vi "Validate Group Time.vi"(0 "Group time":u8) -> (2 "Group Time":u16, 3 "Warning":string, 4 "Frequency (Hz)":dbl)   [LabVIEW 2019]
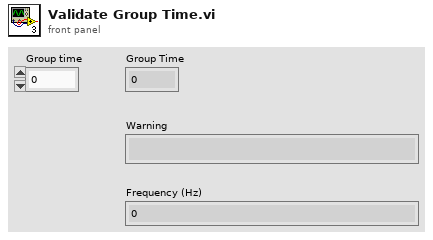
[diagram p1: front panel]
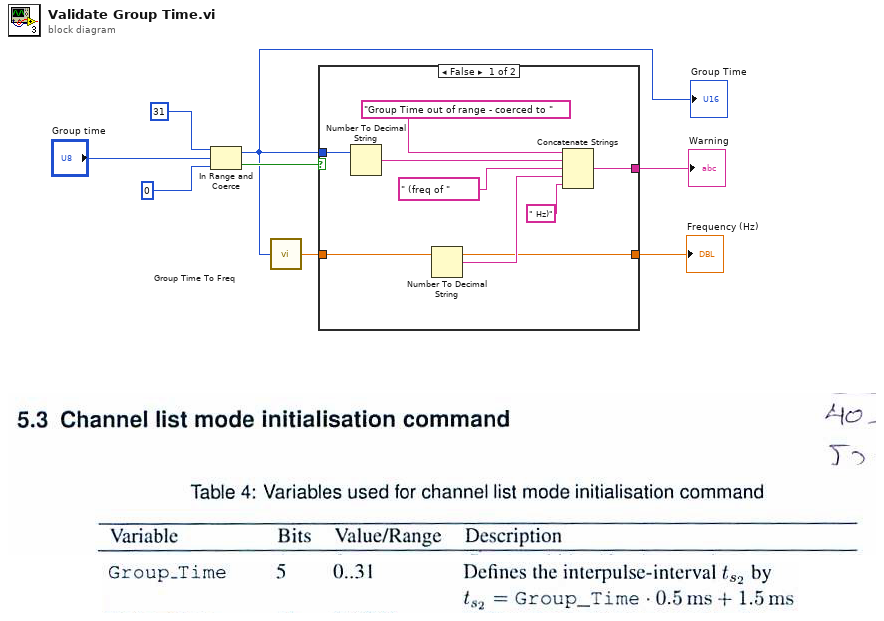
[diagram p0: block diagram]
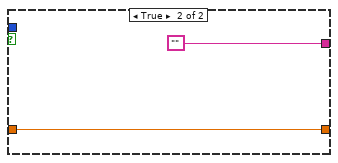
[diagram p2: hidden frame]
diagram:
  n1 = In Range and Coerce(upper limit=u16 31, x="Group time", lower limit=u16 0) -> (coerced(x)=w2:u16, In Range?=w6:bool)
  "Group Time" <- w2
  n2 = call "Group Time To Freq.vi"("Group Time"=w2) -> ("Frequency (Hz)"=w1:dbl)
  n3 = case shown="False" w6 {
    tunnel: w2 -> [w13 _]
    tunnel: [w14 ""] -> w7
    tunnel: w1 -> [w9 w17]
    tunnel: [w9 w17] -> w8
    frame False {
      n4 = Number To Decimal String(number=w13) -> (decimal integer string=w15:string)  [unwired: 1 in]
      n5 = Number To Decimal String(number=w9) -> (decimal integer string=w11:string)  [unwired: 1 in]
      n6 = Concatenate Strings("Group Time out of range - coerced to ", w15, " (freq of " ("string"), w11, " Hz)" ("string")) -> (w14:string)
    }
    frame True {
    }
  }
  "Frequency (Hz)" <- w8
  "Warning" <- w7
